vi "Framework.Get State.vi"(11 "Framework in":refnum<class "Framework.lvclass">) -> (2 "State":refnum<class "Framework State.lvclass">, 3 "Framework out":refnum<class "Framework.lvclass">)   [LabVIEW 2017, in "DSF.Engine.lvlib" / "Framework.lvclass"]
uses:
  Framework.lvclass
  State/Framework State.lvclass
  Framework.lvclass/Framework.ctl
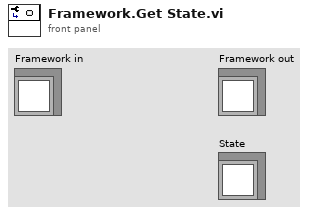
[diagram p1: front panel]
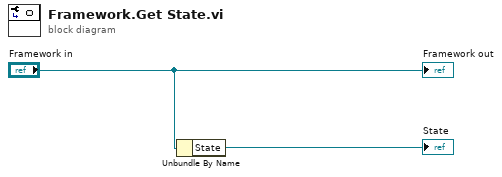
[diagram p0: block diagram]
diagram:
  n1 = Unbundle By Name("Framework in") -> ("State"=→"State":refnum<class "Framework State.lvclass">)
  "Framework out" <- "Framework in"
